vi "CAN_MotorSelect.vi"(0 "Trunk":bool, 1 "Nodes In":refnum<class "sbCANopenBaseClass.lvclass">[](array[class]), 5 "Pelvis":bool, 9 "Pelvis_Moments":bool, 11 "Legs":bool, 12 "Error In":errorcluster[](array[cluster])) -> (3 "maskForTrunkMotors":bool[](array[boolean]), 4 "Nodes Out":refnum<class "sbCANopenBaseClass.lvclass">[](array[class]), 6 "nMotorsCAN":i32, 8 "maskForKneeMotors":bool[](array[boolean]), 10 "CANmotorsuse":bool[](array[boolean]), 14 "Error Out":errorcluster[](array[cluster]), 15 "maskForPelvisMotors":bool[](array[boolean]))   [LabVIEW 2024]
uses:
  <vilib>/addons/Maxon Motor/EPOS2 CANopen/CANopen/sbCANopenBaseClass.lvclass
panel:
  in  "Empty Error":errorcluster[](array[cluster])
  in  "Empty Nodes":refnum<class "sbCANopenBaseClass.lvclass">[](array[class])
  # "Motor Order \n(Trunk, Pelvis, Pelvis_M, Leg)\n3\n6\n9\n12\n2\n7\n8\n13\n4\n5\n10\n11\n1\n14"
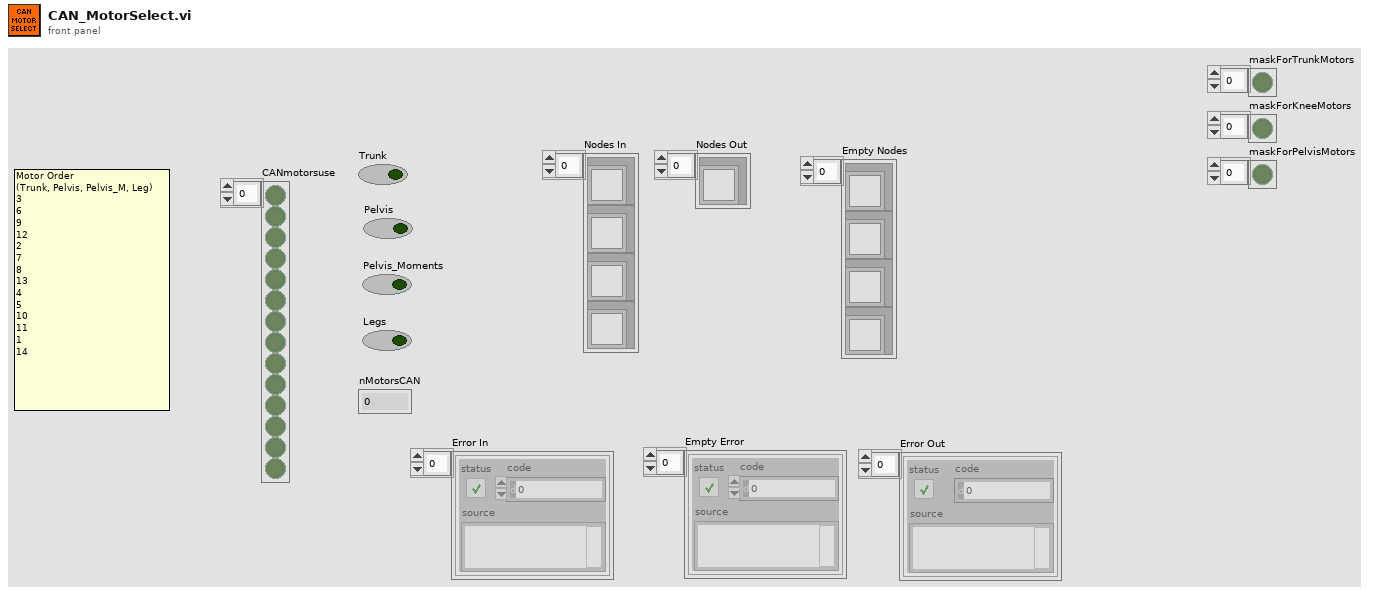
[diagram p1: front panel]
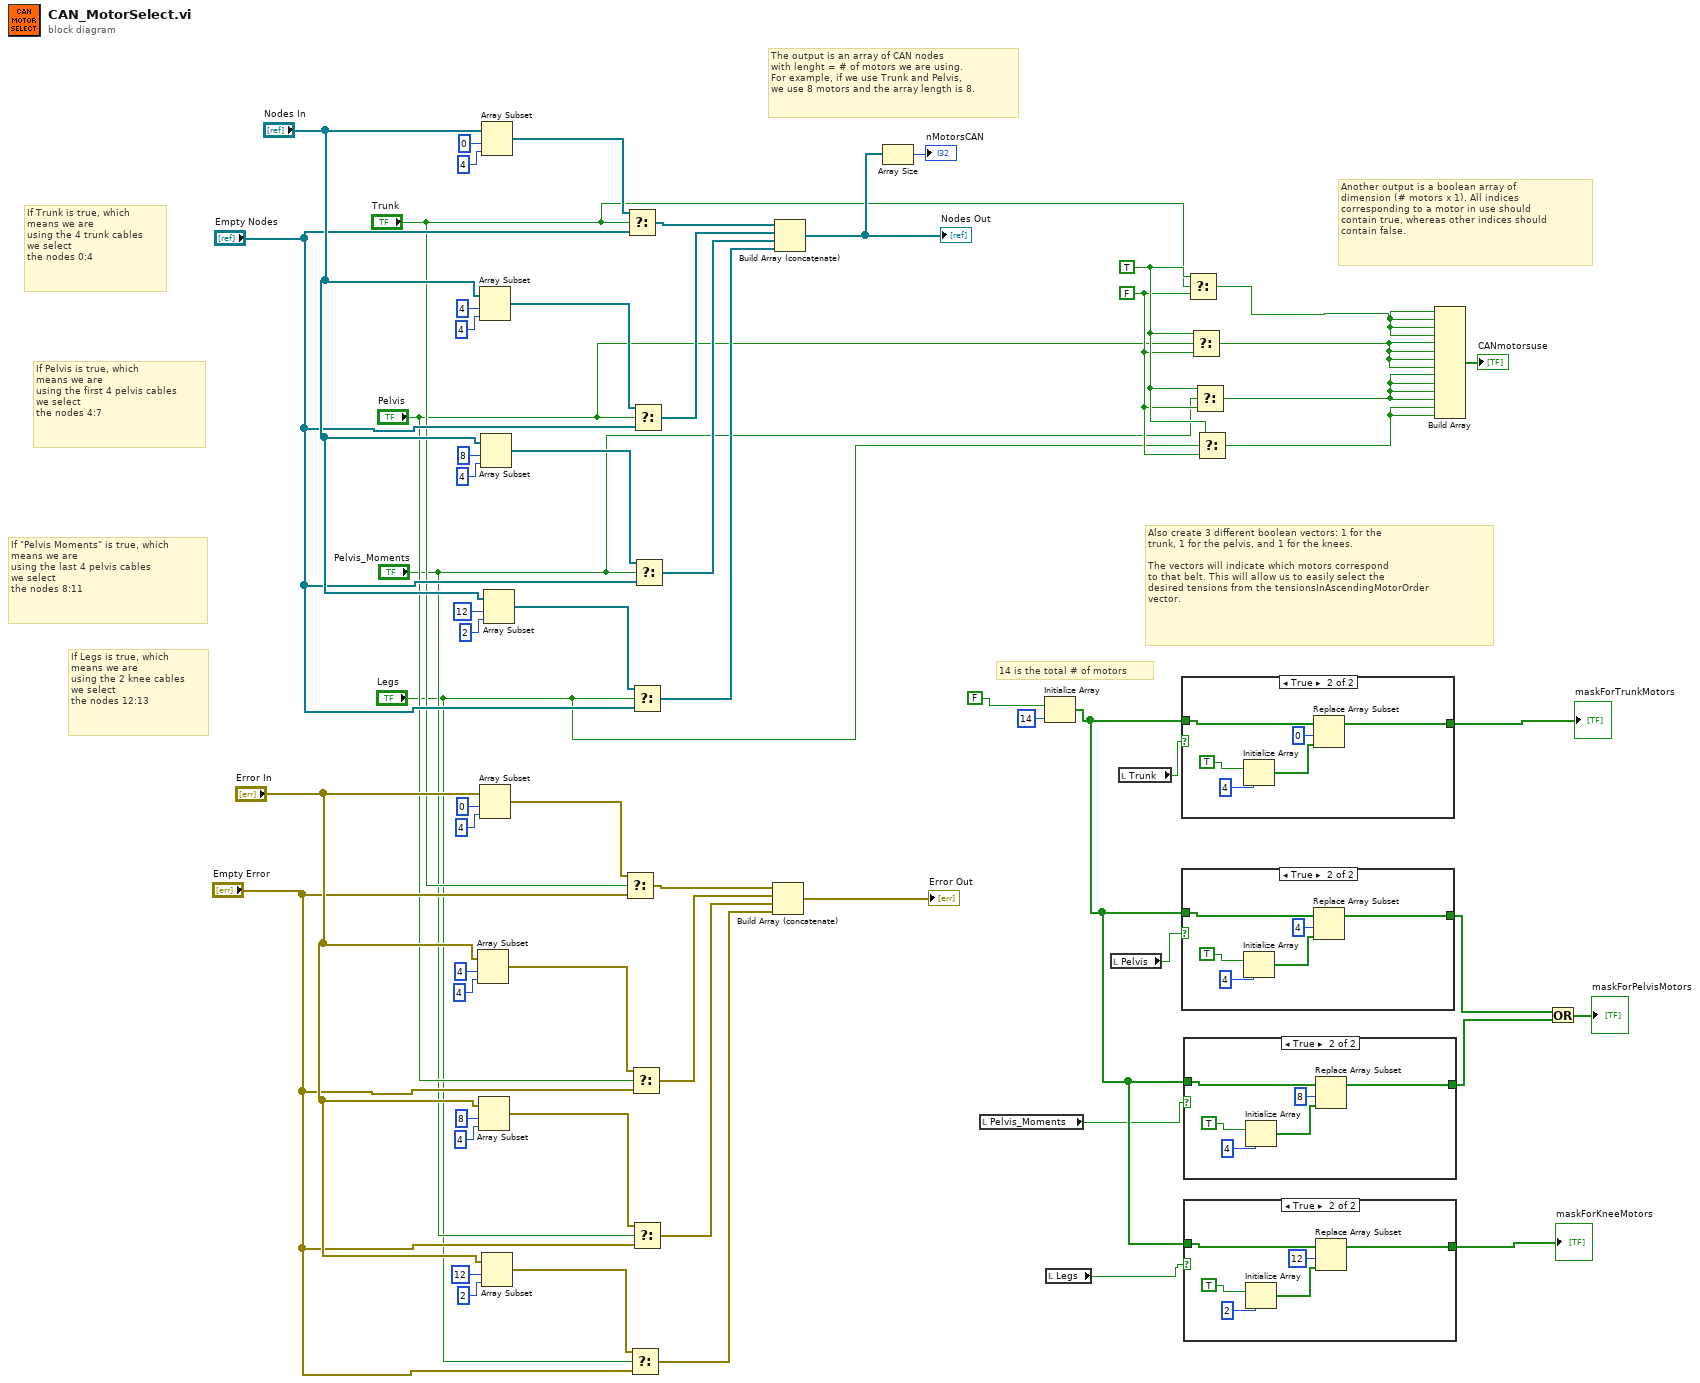
[diagram p0: block diagram]
diagram:
  w22 = FALSE
  w23 = TRUE
  # "14 is the total # of motors"
  # "Also create 3 different boolean vectors: 1 for the \ntrunk, 1 for the pelvis, and 1 for the knees. \n\nThe vectors will indicate which motors correspond \nto that belt. This will allow us to easily select the \ndesired tensions from the tensionsInAscendingMotorOrder\nvector."
  # "Another output is a boolean array of \ndimension (# motors x 1). All indices\ncorresponding to a motor in use should \ncontain true, whereas other indices should \ncontain false."
  # "The output is an array of CAN nodes\nwith lenght = # of motors we are using. \nFor example, if we use Trunk and Pelvis, \nwe use 8 motors and the array length is 8."
  # "If Legs is true, which \nmeans we are \nusing the 2 knee cables\nwe select\nthe nodes 12:13"
  # "If \"Pelvis Moments\" is true, which \nmeans we are \nusing the last 4 pelvis cables\nwe select\nthe nodes 8:11"
  # "If Pelvis is true, which \nmeans we are \nusing the first 4 pelvis cables\nwe select\nthe nodes 4:7"
  # "If Trunk is true, which \nmeans we are \nusing the 4 trunk cables\nwe select\nthe nodes 0:4"
  n1 = Array Subset(array="Error In", index=4, length=4) -> (w32:errorcluster[])
  n2 = Array Subset(array="Error In", index=8, length=4) -> (w33:errorcluster[])
  n3 = Array Subset(array="Nodes In", index=4, length=4) -> (w48:refnum<class "sbCANopenBaseClass.lvclass">[])
  n4 = Array Subset(array="Error In", index=0, length=4) -> (w42:errorcluster[])
  n5 = Array Subset(array="Nodes In", index=8, length=4) -> (w49:refnum<class "sbCANopenBaseClass.lvclass">[])
  n6 = Array Subset(array="Nodes In", index=0, length=4) -> (w60:refnum<class "sbCANopenBaseClass.lvclass">[])
  n7 = Array Subset(array="Error In", index=12, length=2) -> (w34:errorcluster[])
  n8 = Array Subset(array="Nodes In", index=12, length=2) -> (w50:refnum<class "sbCANopenBaseClass.lvclass">[])
  n9 = Select(t=w42, s="Trunk", f="Empty Error") -> (s? t:f=w41:errorcluster[])
  n10 = Select(t=w60, s="Trunk", f="Empty Nodes") -> (s? t:f=w59:refnum<class "sbCANopenBaseClass.lvclass">[])
  n11 = Select(t=w34, s="Legs", f="Empty Error") -> (s? t:f=w29:errorcluster[])
  n12 = Select(t=w32, s="Pelvis", f="Empty Error") -> (s? t:f=w31:errorcluster[])
  n13 = Select(t=w50, s="Legs", f="Empty Nodes") -> (s? t:f=w45:refnum<class "sbCANopenBaseClass.lvclass">[])
  n14 = Select(t=w33, s="Pelvis_Moments", f="Empty Error") -> (s? t:f=w30:errorcluster[])
  n15 = Select(t=w48, s="Pelvis", f="Empty Nodes") -> (s? t:f=w47:refnum<class "sbCANopenBaseClass.lvclass">[])
  n16 = Select(t=w49, s="Pelvis_Moments", f="Empty Nodes") -> (s? t:f=w46:refnum<class "sbCANopenBaseClass.lvclass">[])
  n17 = Build Array (concatenate)(w41, w31, w30, w29) -> (→"Error Out":errorcluster[])
  n18 = Build Array (concatenate)(w59, w47, w46, w45) -> (w25:refnum<class "sbCANopenBaseClass.lvclass">[])
  "Nodes Out" <- w25
  n19 = Array Size(array=w25) -> (size(s)=→"nMotorsCAN":i32)
  n20 = local read "Pelvis_Moments"() -> (w6:bool)
  n21 = Initialize Array(FALSE, 14 ("dimension size")) -> (w8:bool[])
  n22 = local read "Legs"() -> (w5:bool)
  n23 = local read "Pelvis"() -> (w7:bool)
  n24 = local read "Trunk"() -> (w9:bool)
  n25 = case shown="True" w9 {
    tunnel: w8 -> [w63 w69]
    tunnel: [w63 w64] -> w10
    frame False {
    }
    frame True {
      n26 = Initialize Array(TRUE, 4 ("dimension size")) -> (w66:bool[])
      n27 = Replace Array Subset(array=w69, new element=w66, index=0) -> (w64:bool[])
    }
  }
  "maskForTrunkMotors" <- w10
  n28 = case shown="True" w7 {
    tunnel: w8 -> [w70 w76]
    tunnel: [w70 w71] -> w3
    frame False {
    }
    frame True {
      n29 = Initialize Array(TRUE, 4 ("dimension size")) -> (w73:bool[])
      n30 = Replace Array Subset(array=w76, new element=w73, index=4) -> (w71:bool[])
    }
  }
  n31 = case shown="True" w6 {
    tunnel: w8 -> [w77 w83]
    tunnel: [w77 w78] -> w2
    frame False {
    }
    frame True {
      n32 = Initialize Array(TRUE, 4 ("dimension size")) -> (w80:bool[])
      n33 = Replace Array Subset(array=w83, new element=w80, index=8) -> (w78:bool[])
    }
  }
  n34 = case shown="True" w5 {
    tunnel: w8 -> [w84 w90]
    tunnel: [w84 w85] -> w4
    frame False {
    }
    frame True {
      n35 = Initialize Array(TRUE, 2 ("dimension size")) -> (w87:bool[])
      n36 = Replace Array Subset(array=w90, new element=w87, index=12) -> (w85:bool[])
    }
  }
  "maskForKneeMotors" <- w4
  n37 = Select(t=w23, s="Trunk", f=w22) -> (s? t:f=w21:bool)
  n38 = Select(t=w23, s="Pelvis", f=w22) -> (s? t:f=w20:bool)
  n39 = Select(t=w23, s="Pelvis_Moments", f=w22) -> (s? t:f=w19:bool)
  n40 = Select(t=w23, s="Legs", f=w22) -> (s? t:f=w13:bool)
  n41 = Build Array(w21, w21, w21, w21, w20, w20, w20, w20, w19, w19, w19, w19, w13, w13) -> (→"CANmotorsuse":bool[])
  n42 = Or(x=w3, y=w2) -> (x .or. y?=→"maskForPelvisMotors":bool[])
